vi "UMLEditor printHtmlFile.vi"(0 "Report Path":path, 11 "error in (no error)":errorcluster) -> (15 "error out":errorcluster)   [LabVIEW 2016]
doc: "This VI shows a report using IE as an ActiveX-component"
panel:
  in  "SHDocVw.IWebBrowser2":refnum<k7>(container)
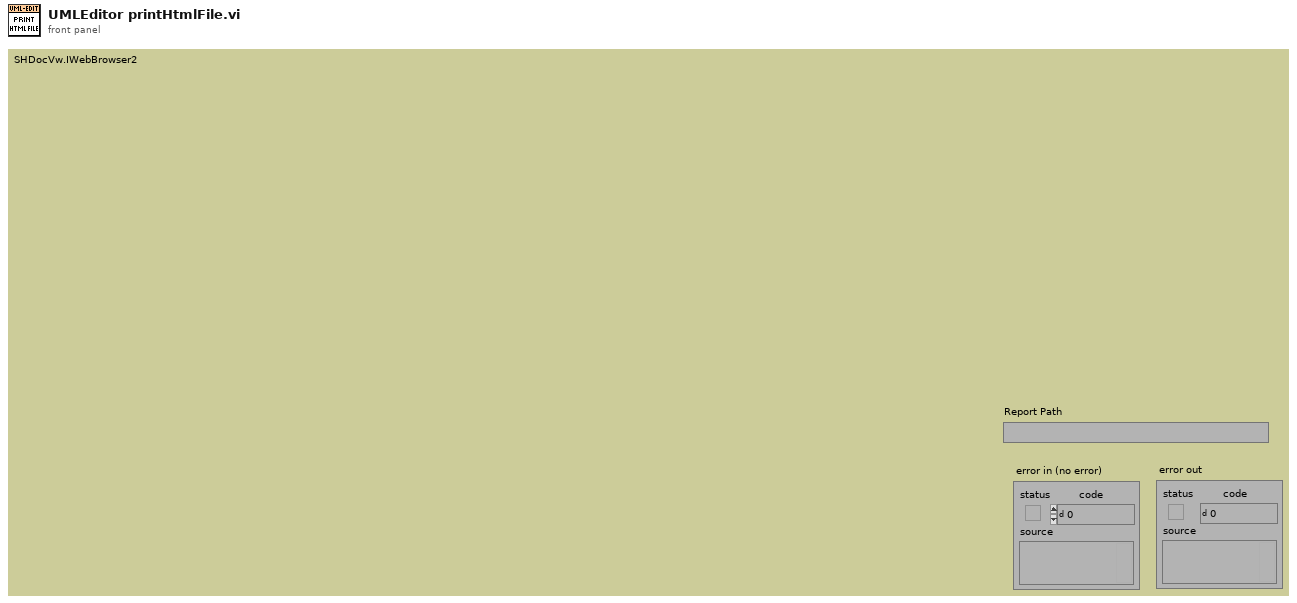
[diagram p1: front panel]
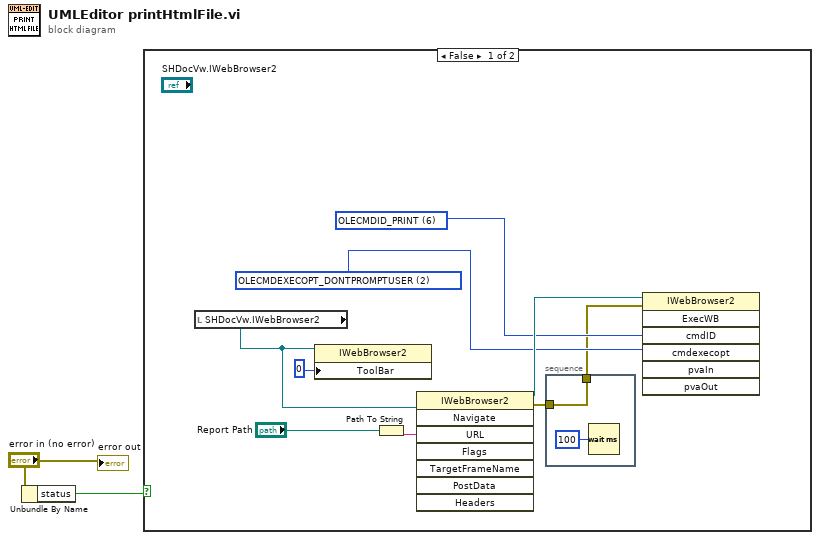
[diagram p0: block diagram]
diagram:
  n1 = Unbundle By Name("error in (no error)") -> ("status"=w1:bool)
  n2 = case shown="False" w1 {
    frame False {
      w5 = 2 items=["OLECMDEXECOPT_DODEFAULT", "OLECMDEXECOPT_PROMPTUSER", "OLECMDEXECOPT_DONTPROMPTUSER", "OLECMDEXECOPT_SHOWHELP"] ("cmdexecopt")
      w9 = 6 items=["OLECMDID_OPEN"=1, "OLECMDID_NEW"=2, "OLECMDID_SAVE"=3, "OLECMDID_SAVEAS"=4, "OLECMDID_SAVECOPYAS"=5, "OLECMDID_PRINT"=6, "OLECMDID_PRINTPREVIEW"=7, "OLECMDID_PAGESETUP"=8, "OLECMDID_SPELL"=9, "OLECMDID_PROPERTIES"=10, "OLECMDID_CUT"=11, "OLECMDID_COPY"=12, "OLECMDID_PASTE"=13, "OLECMDID_PASTESPECIAL"=14, "OLECMDID_UNDO"=15, "OLECMDID_REDO"=16, "OLECMDID_SELECTALL"=17, "OLECMDID_CLEARSELECTION"=18, "OLECMDID_ZOOM"=19, "OLECMDID_GETZOOMRANGE"=20, "OLECMDID_UPDATECOMMANDS"=21, "OLECMDID_REFRESH"=22, "OLECMDID_STOP"=23, "OLECMDID_HIDETOOLBARS"=24, "OLECMDID_SETPROGRESSMAX"=25, "OLECMDID_SETPROGRESSPOS"=26, "OLECMDID_SETPROGRESSTEXT"=27, "OLECMDID_SETTITLE"=28, "OLECMDID_SETDOWNLOADSTATE"=29, "OLECMDID_STOPDOWNLOAD"=30, "OLECMDID_ONTOOLBARACTIVATED"=31, "OLECMDID_FIND"=32, "OLECMDID_DELETE"=33, "OLECMDID_HTTPEQUIV"=34, "OLECMDID_HTTPEQUIV_DONE"=35, "OLECMDID_ENABLE_INTERACTION"=36, "OLECMDID_ONUNLOAD"=37, "OLECMDID_PROPERTYBAG2"=38, "OLECMDID_PREREFRESH"=39] ("cmdID")
      n3 = local read "SHDocVw.IWebBrowser2"() -> (w6:refnum<k7>)
      n4 = property class="IWebBrowser2"(reference=w6, "ToolBar"=0) -> ()  [unwired: 1 in, 2 out]
      n5 = Path To String(path="Report Path") -> (string=w8:string)
      n6 = invoke class="IWebBrowser2" method="Navigate"(reference=w6, "URL"=w8) -> (reference out=w10:refnum<k7>, error out=w3:errorcluster)  [unwired: 6 in, 6 out]
      n7 = stacked-sequence {
        tunnel: [w12] -> w4
        tunnel: w3 -> [w12]
        frame #0 {
          n8 = Wait (ms)(milliseconds to wait=u32 100) -> ()  [unwired: 1 out]
        }
      }
      n9 = invoke class="IWebBrowser2" method="ExecWB"(reference=w10, error in=w4, "cmdID"=w9, "cmdexecopt"=w5) -> ()  [unwired: 3 in, 7 out]
    }
    frame True {
    }
  }
  "error out" <- "error in (no error)"
